vi "Check Alignment.vi"(8 "Current State":T1=enum."Turn Tote Right", 10 "Right Pot":dbl, 11 "Left Pot":dbl) -> (3 "State Output":T1=enum."Turn Tote Right")   [LabVIEW 2014]
uses:
  Common Code/Inner Roller States.ctl
  Robot Global Data.vi
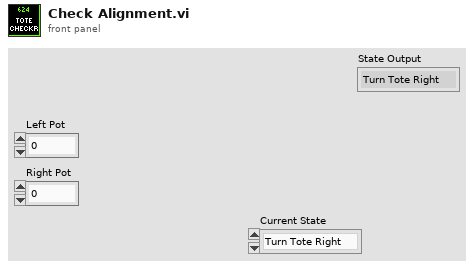
[diagram p1: front panel]
types:
  T1 = typedef "Inner Roller States.ctl" = enum16{"Acquire Tote", "Absorb Tote", "Turn Tote Right", "Turn Tote Left"}
  T2 = typedef "Dashboard Control Data.ctl" = cluster{"Cam Exposure":dbl, "Go to angle":dbl, "Steer PID Gains":cluster{"proportional gain (Kc)":dbl, "integral time (Ti, min)":dbl, "derivative time (Td, min)":dbl}, "Steer PID output Range":cluster{"output high":dbl, "output low":dbl}, "Pressure m \nValue":dbl, "Pressure b \nValue":dbl, "Strafe Timer\nWait":dbl, "Roller Command Cluster ":T3, "Elevator":T4, "Strafe Correct min X":dbl, "IMU Enable":bool, "Encoder Control":T6}
  T3 = typedef "Roller Control.ctl" = cluster{"Left Roller Speed":dbl, "Right Roller Speed":dbl, "Left Roller Speed Back":dbl, "Right Roller Speed Back":dbl, "Roller Align Decide Limit":u32, "Left Roller Speed Unload":dbl, "Right Roller Speed Unload":dbl, "Ping Dist Difference":dbl, "Ping In Dist":dbl, "Right Pot 0":dbl, "Pot Threshold":dbl, "Left Pot 0":dbl, "Manual 0s?":bool, "Right Pot Scale":dbl, "Left Pot Scale":dbl, "0 wait time":i32, "Reset?":bool}
  T4 = typedef "Elevator DB Control.ctl" = cluster{"PID Output Range":cluster{"output high":dbl, "output low":dbl}, "PID gains":cluster{"proportional gain (Kc)":dbl, "integral time (Ti, min)":dbl, "derivative time (Td, min)":dbl}, "Height Tolerance":dbl, " Encoder Constant":dbl, "Safe Mode Max Speed":dbl, "Eject Time":dbl, "Encoder Filter?":bool, "Zeroing Speed":dbl, "Presets":T5}
  T5 = typedef "Elevator Presets.ctl" = cluster{"Hold Tote":dbl, "Hold Trashcan":dbl, "Pickup 2 w/ Tote":dbl, "Pickup 2 w/ Trashcan":dbl, "Pickup 3 w/ Tote":dbl, "Pickup 3 w/ Trashcan":dbl, "Bottom":dbl, "Pickup 1 w/ Tote":dbl, "Pickup Trashcan":dbl, "Pickup 1 w/ Trashcan":dbl, "Eject":dbl}
  T6 = typedef "Encoder Control.ctl" = cluster{"Left Tick Constant":dbl, "Right Tick Constant":dbl, "Center Tick Constant":dbl, "Reset?":bool}
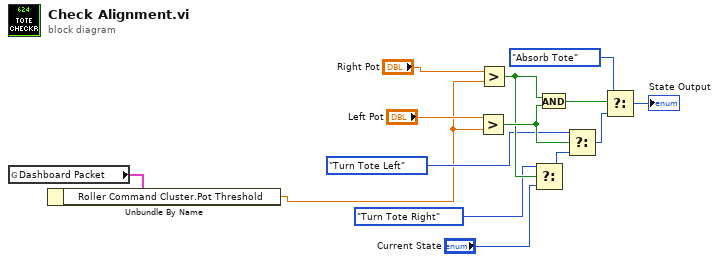
[diagram p0: block diagram]
diagram:
  n1 = global read "Robot Global Data.vi" "Dashboard Packet"() -> (w2:T2)
  n2 = Unbundle By Name(w2) -> ("Roller Command Cluster.Pot Threshold"=w1:dbl)
  n3 = Greater?(x="Left Pot", y=w1) -> (0:w11:bool)
  n4 = Greater?(x="Right Pot", y=w1) -> (0:w10:bool)
  n5 = Select(t=Inner_Roller_States."Turn Tote Right" ("Enum"), s=w10, f="Current State") -> (s? t:f=w12:T1)
  n6 = And(x=w10, y=w11) -> (x .and. y?=w14:bool)
  n7 = Select(t=Inner_Roller_States."Turn Tote Left" ("Enum"), s=w11, f=w12) -> (s? t:f=w8:T1)
  n8 = Select(t=Inner_Roller_States."Absorb Tote" ("Enum"), s=w14, f=w8) -> (s? t:f=→"State Output":T1)
